vi "Frame Page.vi"(8 "error in (no error)":errorcluster, 11 "Node Ptr":T2 format="%.0x") -> (0 "error out":errorcluster)   [LabVIEW 2023, in "Protection and Counter Addon System Explorer.lvlib"]
uses:
  Protection and Counter Addon System Explorer.lvlib
  <vilib>/NI VeriStand/Custom Device API/Custom Device Item Ref.ctl
  NationalInstruments.VeriStand.SystemStorageUI
  Types/Event Trigger Type.ctl
  <vilib>/NI VeriStand/UI Controls/Single Node Browser/Net Event Data.ctl
  <vilib>/NI VeriStand/UI Controls/Single Node Browser/Net Event.ctl
  Addon Shared/SubVIs/GUID Lookup.vi
  <vilib>/NI VeriStand/Custom Device API/Custom Device API.lvlib
  <vilib>/NI VeriStand/UI Controls/Single Node Browser/NI_VS UI Single Node Browser.lvlib
  Addon Shared/Protection and Counter Addon Shared.lvlib
panel:
  in  "Start Time Offset (ms)":u32
  in  "Transmit Trigger":T1
  in  "Trigger":refnum<k24>(container)
  in  "Trigger Settings":cluster{"Section Name":string}={"Section Name"="Transmission Trigger"}
  in  "Trigger":refnum<k24>(container)
  in  "Disable Transmission":bool
  in  "Disable Settings":cluster{"Section Name":string}={"Section Name"="Disable Transmission"}
  in  "Description":string
  out "Frame ID":u32 format="%.0x"
  in  "Custom Device Settings":cluster{"Section Name":string}={"Section Name"="Frame Settings"}
  out "Name":string
  in  "SHDocVw.IWebBrowser2":refnum<k7>(container)
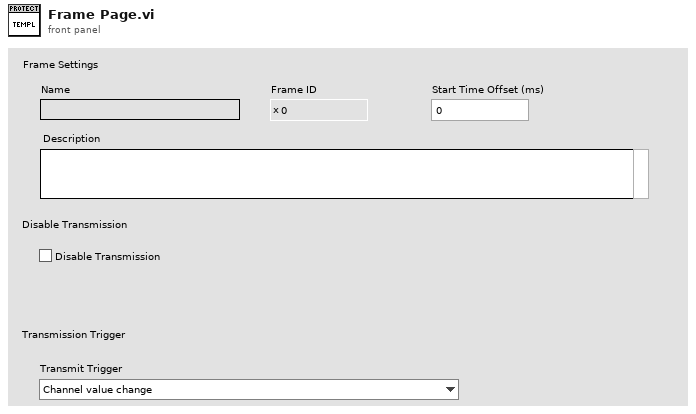
[diagram p1: front panel]
types:
  T1 = typedef "Protection and Counter Addon System Explorer.lvlib/Event Trigger Type.ctl" = enum16{"Channel value change", "Trigger channel (not zero)", "Channel value change or trigger channel (not zero)", "Trigger channel (any value change)", "Channel value change or trigger channel (any value change)"}
  T2 = typedef "Custom Device API.lvlib/Custom Device Item Ref.ctl" = u64
  T3 = cluster{"Trigger":refnum<user-event>, "Transmission":refnum<user-event>}
  T4 = typedef "Protection and Counter Addon System Explorer.lvlib/Frame Settings.ctl" = cluster{"ID":u32, "Disable Transmission":bool, "Disable Transmission Ref":T2, "Transmit Trigger":T1, "Transmit Trigger Ref":T2, "Start Time Offset (ms)":u16}
  T5 = typedef "Custom Device API.lvlib/Custom Device Item Info.ctl" = cluster{"Name":string, "Is Channel":bool, "GUID":string, "Is Waveform":bool}
  T6 = typedef "NI_VS UI Single Node Browser.lvlib/Single Node Browser Ref.ctl" = refnum<k24>
  T7 = typedef "NI_VS UI Single Node Browser.lvlib/Callback Type.ctl" = cluster{"Net Callbacks":refnum<k27>[], "Event":refnum<user-event>}
  T8 = typedef "Custom Device API.lvlib/Custom Device Commands.ctl" = enum16{"Default", "Item renamed", "Shutdown", "Dynamic button pressed"}
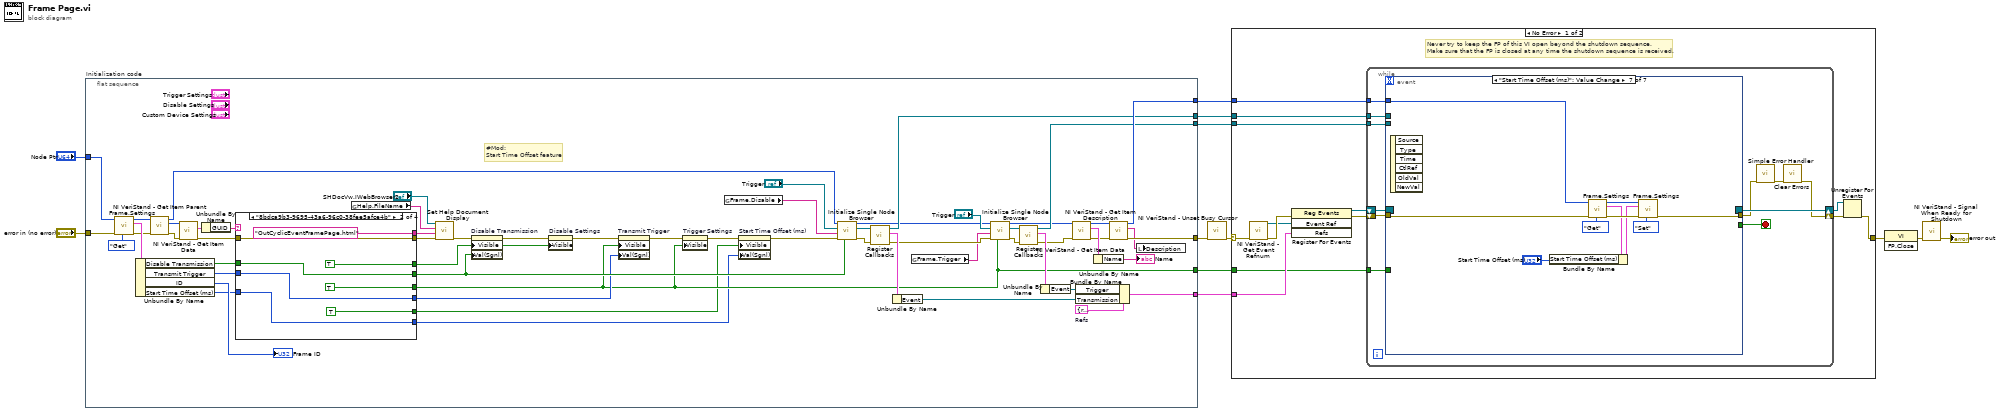
[diagram p0: block diagram]
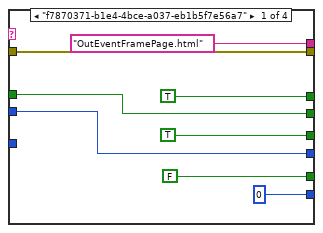
[diagram p2: hidden frame]
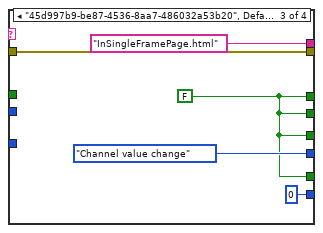
[diagram p3: hidden frame]
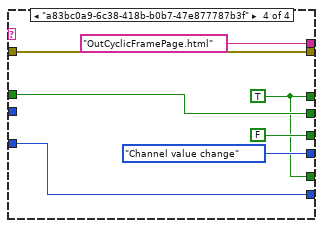
[diagram p4: hidden frame]
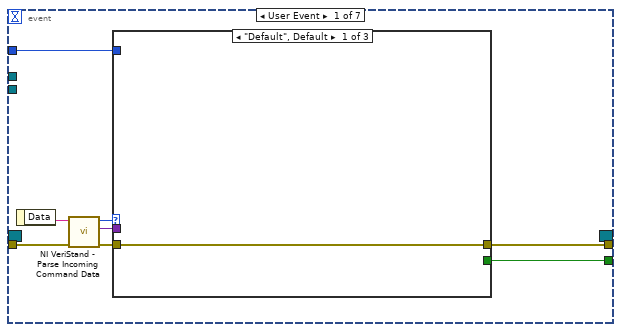
[diagram p5: hidden frame]
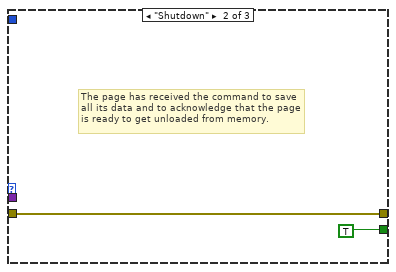
[diagram p6: hidden frame]
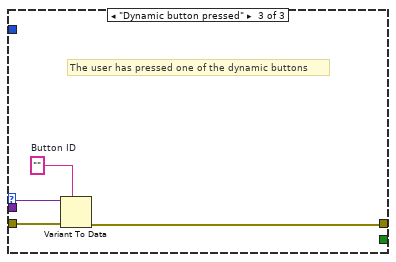
[diagram p7: hidden frame]
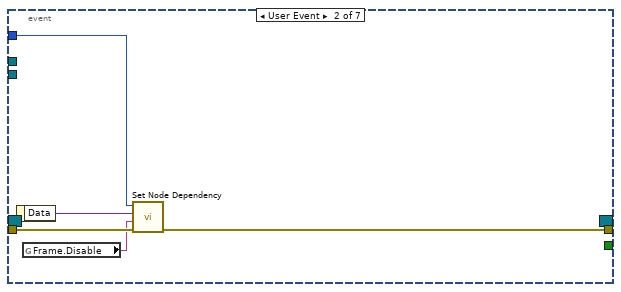
[diagram p8: hidden frame]
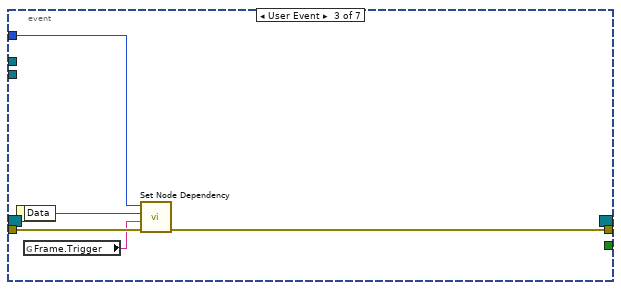
[diagram p9: hidden frame]
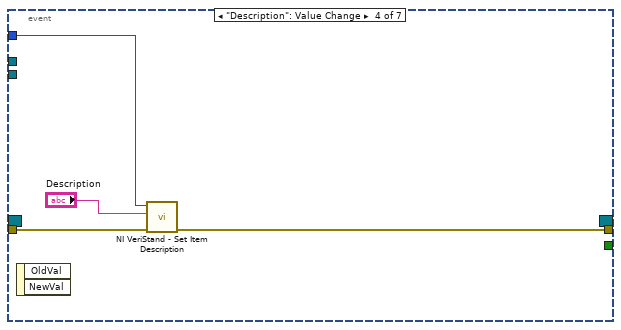
[diagram p10: hidden frame]
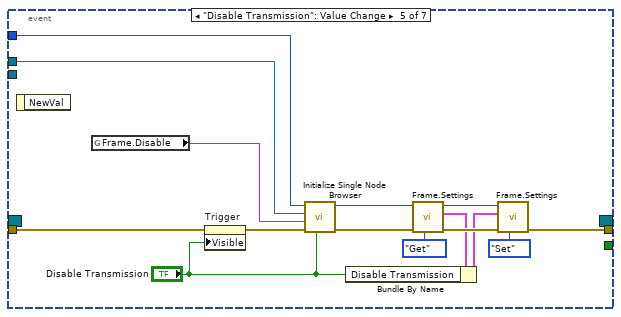
[diagram p11: hidden frame]
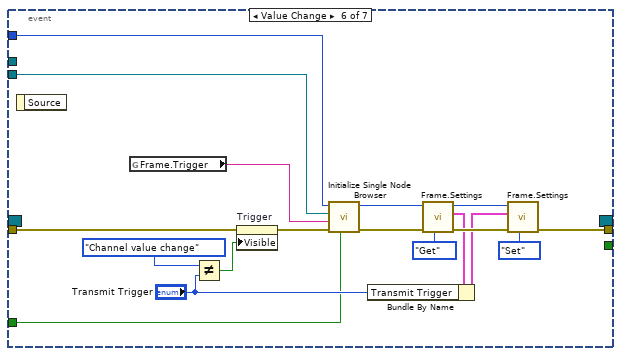
[diagram p12: hidden frame]
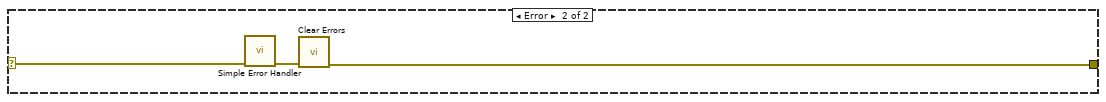
[diagram p13: hidden frame]
diagram:
  n1 = flat-sequence "Initialization code" {
    tunnel: "error in (no error)" -> [w28]
    tunnel: "Node Ptr" -> [w26]
    tunnel: [w66] -> w7
    tunnel: [w64] -> w5
    tunnel: [w48] -> w4
    tunnel: [w50] -> w3
    tunnel: [w40] -> w2
    tunnel: [w21] -> w1
    frame #0 {
      w43 = T3 {"Trigger"=refnum, "Transmission"=refnum}  # Refs
      # "#Mod:\nStart Time Offset feature"
      n2 = call "Frame.Settings.vi"("Action"=enum8{"Get", "Set"}."Get", "error in (no error)"=w28, "Item Ref in"=w26) -> ("error out"=w27:errorcluster, "Frame.Settings"=w32:T4, "Item Ref out"=w25:T2)  [unwired: 6 in]
      n3 = Unbundle By Name(w32) -> ("Disable Transmission"=w24:bool, "Transmit Trigger"=w23:T1, "ID"=→"Frame ID":u32, "Start Time Offset (ms)"=w15:u16)
      n4 = call <vilib>:"NI VeriStand - Get Item Parent.vi"("error in (no error)"=w27, "Item Ref in"=w25) -> ("error out"=w62:errorcluster, "Parent Ref"=w61:T2, "Item Ref out"=w54:T2)  [unwired: 6 in, 1 out]
      n5 = call <vilib>:"NI VeriStand - Get Item Data.vi"("error in (no error)"=w62, "Item Ref in"=w61) -> ("error out"=w58:errorcluster, "Item Info"=w60:T5)  [unwired: 8 out]
      n6 = Unbundle By Name(w60) -> ("GUID"=w59:string)
      n7 = case shown="\"8bdca9b3-9695-43a6-96c0-38fee5afce4b\"" w59 {
        tunnel: ["OutEventFramePage.html" ("HTML File") "OutCyclicEventFramePage.html" ("HTML File") "InSingleFramePage.html" ("HTML File") "OutCyclicFramePage.html" ("HTML File")] -> w70
        tunnel: w58 -> [w78 w86 w91 w98]
        tunnel: [w78 w86 w91 w98] -> w34
        tunnel: [TRUE TRUE w89 w93] -> w51
        tunnel: [w74 w82 w89 w96] -> w36
        tunnel: [TRUE TRUE w89 FALSE] -> w21
        tunnel: [w75 w83 Event_Trigger_Type."Channel value change" ("y") Event_Trigger_Type."Channel value change" ("y")] -> w35
        tunnel: w24 -> [w74 w82 _ w96]
        tunnel: w23 -> [w75 w83 _ _]
        tunnel: w15 -> [_ w80 _ w94]
        tunnel: [u16 0 ("Start Time Offset (ms)") w80 u16 0 ("Start Time Offset (ms)") w94] -> w14
        tunnel: [FALSE TRUE w89 w93] -> w13
        frame "f7870371-b1e4-4bce-a037-eb1b5f7e56a7" {
        }
        frame "8bdca9b3-9695-43a6-96c0-38fee5afce4b" {
        }
        frame "45d997b9-be87-4536-8aa7-486032a53b20", Default {
          w89 = FALSE
        }
        frame "a83bc0a9-6c38-418b-b0b7-47e877787b3f" {
          w93 = TRUE
        }
      }
      n8 = global read "GUID Lookup.vi" "Help.FileName"() -> (w18:string)
      n9 = call "Set Help Document Display.vi"("error in (no error)"=w34, "HTML File"=w70, "Main CHM File"=w18, "SHDocVw.IWebBrowser2"="SHDocVw.IWebBrowser2") -> ("error out"=w33:errorcluster)  [unwired: 7 in]
      n10 = property on="Disable Transmission" class="Bool (strict)"(error in=w33, "Visible"=w51, "Val(Sgnl)"=w36) -> (error out=w57:errorcluster)  [unwired: 1 in, 1 out]
      n11 = property on="Disable Settings" class="Clust (strict)"(error in=w57, "Visible"=w51) -> (error out=w38:errorcluster)  [unwired: 1 in, 1 out]
      n12 = property on="Transmit Trigger" class="Enum (strict)"(error in=w38, "Visible"=w21, "Val(Sgnl)"=w35) -> (error out=w37:errorcluster)  [unwired: 1 in, 1 out]
      n13 = property on="Trigger Settings" class="Clust (strict)"(error in=w37, "Visible"=w21) -> (error out=w17:errorcluster)  [unwired: 1 in, 1 out]
      n14 = global read "GUID Lookup.vi" "Frame.Disable"() -> (w20:string)
      n15 = property on="Start Time Offset (ms)" class="DigNum (strict)"(error in=w17, "Visible"=w13, "Val(Sgnl)"=w14) -> (error out=w16:errorcluster)  [unwired: 1 in, 1 out]
      n16 = call "Initialize Single Node Browser.vi"("Use Channel?"=w36, "error in (no error)"=w16, "NodeName"=w20, "Browser Ref 2"="Trigger", "Item Ref in"=w54) -> ("error out"=w56:errorcluster, "Browser Ref"=w55:T6, "Item Ref out"=w39:T2)  [unwired: 4 in]
      n17 = call <vilib>:"Register Callbacks.vi"("error in (no error)"=w56, "Single Node Browser"=w55) -> ("error out"=w44:errorcluster, "Callbacks"=w53:T7, "Single Node Browser dup"=w50:T6)  [unwired: 7 in]
      n18 = Unbundle By Name(w53) -> ("Event"=w49:refnum<user-event>)
      n19 = global read "GUID Lookup.vi" "Frame.Trigger"() -> (w19:string)
      n20 = call "Initialize Single Node Browser.vi"("Use Channel?"=w21, "error in (no error)"=w44, "NodeName"=w19, "Browser Ref 2"="Trigger", "Item Ref in"=w39) -> ("error out"=w45:errorcluster, "Browser Ref"=w46:T6, "Item Ref out"=w29:T2)  [unwired: 4 in]
      n21 = call <vilib>:"Register Callbacks.vi"("error in (no error)"=w45, "Single Node Browser"=w46) -> ("error out"=w30:errorcluster, "Callbacks"=w47:T7, "Single Node Browser dup"=w40:T6)  [unwired: 7 in]
      n22 = Unbundle By Name(w47) -> ("Event"=w42:refnum<user-event>)
      n23 = call <vilib>:"NI VeriStand - Get Item Data.vi"("error in (no error)"=w30, "Item Ref in"=w29) -> ("error out"=w67:errorcluster, "Item Info"=w69:T5, "Item Ref out"=w65:T2)  [unwired: 7 out]
      n24 = Bundle By Name(cluster=w43, "Trigger"=w42, "Transmission"=w49) -> (w48:T3)
      n25 = Unbundle By Name(w69) -> ("Name"=→"Name":string)
      n26 = call <vilib>:"NI VeriStand - Get Item Description.vi"("error in (no error)"=w67, "Item Ref in"=w65) -> ("error out"=w66:errorcluster, "Description"=w63:string, "Item Ref out"=w64:T2)  [unwired: 7 out]
      n27 = local write "Description"(w63) -> ()
    }
  }
  n28 = call <vilib>:"NI VeriStand - Unset Busy Cursor.vi"("error in (no error)"=w7) -> ("error out"=w9:errorcluster)  [unwired: 10 out]
  n29 = case shown="No Error" w9 {
    selector: w9 -> [w104 w198]
    tunnel: [w109 w196] -> w12
    tunnel: w5 -> [w105 _]
    tunnel: w4 -> [w103 _]
    tunnel: w3 -> [w102 _]
    tunnel: w2 -> [w101 _]
    tunnel: w1 -> [w100 _]
    frame No Error {
      # "Never try to keep the FP of this VI open beyond the shutdown sequence.\nMake sure that the FP is closed at any time the shutdown sequence is received."
      n30 = call <vilib>:"NI VeriStand - Get Event Refnum.vi"("error in (no error)"=w104) -> ("error out"=w112:errorcluster, "Event Ref"=w108:refnum<user-event>)  [unwired: 9 out]
      n31 = register-events(error in=w112, w108, w103) -> (reference out=w106:refnum<event-registration>, error out=w107:errorcluster)  [unwired: 1 in]
      n32 = while {
        tunnel: w105 -> [w119]
        shift-right: [w116] -> w110
        shift-left: w107 -> [w122]
        shift-right: [w123] -> w111
        shift-left: w106 -> [w121]
        tunnel: w102 -> [w115]
        tunnel: w101 -> [w114]
        tunnel: w100 -> [w113]
        stop <- w120 stop-if-true
        n33 = event shown="[6] \"Start Time Offset (ms)\": Value Change" {
          selector: w121 -> [_ _ _ _ _ _ _]
          dyn-events: [_ _ _ _ _ _ _] -> w123
          timeout: _ -> [_ _ _ _ _ _ _]
          tunnel: w122 -> [w131 w141 w146 w152 w167 w185 w189]
          tunnel: [w127 _ _ _ _ _ _] -> w120
          tunnel: [w126 w140 w145 w151 w158 w172 w190] -> w118
          tunnel: w119 -> [w125 w142 w147 w150 w165 w184 w191]
          tunnel: w115 -> [_ _ _ _ w166 _ _]
          tunnel: w114 -> [_ _ _ _ _ w180 _]
          tunnel: w113 -> [_ _ _ _ _ w170 _]
          event User Event {
            n34 = event-data() -> ("Data"=w130:string)  [unwired: 1 out]
            n35 = call <vilib>:"NI VeriStand - Parse Incoming Command Data.vi"("error in (no error)"=w131, "Incoming data"=w130) -> ("error out"=w129:errorcluster, "Outgoing data"=w124:variant, "Action"=w128:T8)  [unwired: 7 out]
            n36 = case shown="\"Default\", Default" w128 {
              tunnel: w129 -> [w132 w133 w138]
              tunnel: [_ TRUE _] -> w127
              tunnel: [w132 w133 w135] -> w126
              tunnel: w125 -> [_ _ _]
              tunnel: w124 -> [_ _ w137]
              frame "Default", Default {
              }
              frame "Shutdown" {
                # "The page has received the command to save all its data and to acknowledge that the page is ready to get unloaded from memory."
              }
              frame "Dynamic button pressed" {
                w136 = ""  # Button ID
                # "The user has pressed one of the dynamic buttons"
                n37 = Variant To Data(error in=w138, type=w136, Variant=w137) -> (error out=w135:errorcluster)  [unwired: 1 out]
              }
            }
          }
          event User Event {
            n38 = event-data() -> ("Data"=w143:variant)  [unwired: 1 out]
            n39 = global read "GUID Lookup.vi" "Frame.Disable"() -> (w139:string)
            n40 = call "Set Node Dependency.vi"("error in (no error)"=w141, "NodeName"=w139, "Data"=w143, "Item Ref in"=w142) -> ("error out"=w140:errorcluster)  [unwired: 6 in, 1 out]
          }
          event User Event {
            n41 = event-data() -> ("Data"=w148:variant)  [unwired: 1 out]
            n42 = global read "GUID Lookup.vi" "Frame.Trigger"() -> (w144:string)
            n43 = call "Set Node Dependency.vi"("error in (no error)"=w146, "NodeName"=w144, "Data"=w148, "Item Ref in"=w147) -> ("error out"=w145:errorcluster)  [unwired: 6 in, 1 out]
          }
          event "Description": Value Change {
            n44 = event-data() -> ()  [unwired: 3 out]
            n45 = call <vilib>:"NI VeriStand - Set Item Description.vi"("error in (no error)"=w152, "Description"="Description", "Item Ref in"=w150) -> ("error out"=w151:errorcluster)  [unwired: 8 out]
          }
          event "Disable Transmission": Value Change {
            n46 = event-data() -> ()  [unwired: 2 out]
            n47 = global read "GUID Lookup.vi" "Frame.Disable"() -> (w153:string)
            n48 = property on="Trigger" class="AXCont"(error in=w167, "Visible"="Disable Transmission") -> (error out=w164:errorcluster)  [unwired: 1 in, 1 out]
            n49 = call "Initialize Single Node Browser.vi"("Use Channel?"="Disable Transmission", "error in (no error)"=w164, "NodeName"=w153, "Browser Ref 2"=w166, "Item Ref in"=w165) -> ("error out"=w161:errorcluster, "Item Ref out"=w162:T2)  [unwired: 4 in, 1 out]
            n50 = call "Frame.Settings.vi"("Action"=enum8{"Get", "Set"}."Get", "error in (no error)"=w161, "Item Ref in"=w162) -> ("error out"=w159:errorcluster, "Frame.Settings"=w156:T4, "Item Ref out"=w157:T2)  [unwired: 6 in]
            n51 = Bundle By Name(cluster=w156, "Disable Transmission"="Disable Transmission") -> (w154:T4)
            n52 = call "Frame.Settings.vi"("Action"=enum8{"Get", "Set"}."Set", "error in (no error)"=w159, "Frame.Settings"=w154, "Item Ref in"=w157) -> ("error out"=w158:errorcluster)  [unwired: 5 in, 2 out]
          }
          event Value Change {
            n53 = event-data() -> ()  [unwired: 2 out]
            n54 = global read "GUID Lookup.vi" "Frame.Trigger"() -> (w168:string)
            n55 = Not Equal?(x=Event_Trigger_Type."Channel value change" ("y"), y="Transmit Trigger") -> (x != y?=w181:bool)
            n56 = property on="Trigger" class="AXCont"(error in=w185, "Visible"=w181) -> (error out=w183:errorcluster)  [unwired: 1 in, 1 out]
            n57 = call "Initialize Single Node Browser.vi"("Use Channel?"=w170, "error in (no error)"=w183, "NodeName"=w168, "Browser Ref 2"=w180, "Item Ref in"=w184) -> ("error out"=w173:errorcluster, "Item Ref out"=w171:T2)  [unwired: 4 in, 1 out]
            n58 = call "Frame.Settings.vi"("Action"=enum8{"Get", "Set"}."Get", "error in (no error)"=w173, "Item Ref in"=w171) -> ("error out"=w177:errorcluster, "Frame.Settings"=w175:T4, "Item Ref out"=w176:T2)  [unwired: 6 in]
            n59 = Bundle By Name(cluster=w175, "Transmit Trigger"="Transmit Trigger") -> (w169:T4)
            n60 = call "Frame.Settings.vi"("Action"=enum8{"Get", "Set"}."Set", "error in (no error)"=w177, "Frame.Settings"=w169, "Item Ref in"=w176) -> ("error out"=w172:errorcluster)  [unwired: 5 in, 2 out]
          }
          event "Start Time Offset (ms)": Value Change {
            n61 = event-data() -> ()  [unwired: 7 out]
            n62 = call "Frame.Settings.vi"("Action"=enum8{"Get", "Set"}."Get", "error in (no error)"=w189, "Item Ref in"=w191) -> ("error out"=w193:errorcluster, "Frame.Settings"=w188:T4, "Item Ref out"=w192:T2)  [unwired: 6 in]
            n63 = Bundle By Name(cluster=w188, "Start Time Offset (ms)"="Start Time Offset (ms)") -> (w187:T4)
            n64 = call "Frame.Settings.vi"("Action"=enum8{"Get", "Set"}."Set", "error in (no error)"=w193, "Frame.Settings"=w187, "Item Ref in"=w192) -> ("error out"=w190:errorcluster)  [unwired: 5 in, 2 out]
          }
        }
        n65 = call <vilib>:"Simple Error Handler.vi"("error in (no error)"=w118) -> ("error out"=w117:errorcluster)  [unwired: 1 in, 7 out]
        n66 = call <vilib>:"Clear Errors.vi"("error in (no error)"=w117) -> ("error out"=w116:errorcluster)  [unwired: 1 in, 5 out]
      }
      n67 = Unregister For Events(event registration refnum=w111, error in=w110) -> (error out=w109:errorcluster)
    }
    frame Error {
      n68 = call <vilib>:"Simple Error Handler.vi"("error in (no error)"=w198) -> ("error out"=w197:errorcluster)  [unwired: 1 in, 7 out]
      n69 = call <vilib>:"Clear Errors.vi"("error in (no error)"=w197) -> ("error out"=w196:errorcluster)  [unwired: 1 in, 5 out]
    }
  }
  n70 = invoke class="VI" method="FP.Close"(error in=w12) -> (error out=w11:errorcluster)  [unwired: 2 in, 2 out]
  n71 = call <vilib>:"NI VeriStand - Signal When Ready for Shutdown.vi"("error in (no error)"=w11) -> ("error out"=→"error out":errorcluster)  [unwired: 10 out]
